vi "XIPIN_Aurora_8B10B_11_0.vi"   [LabVIEW 2017]
doc: "Customizable multi-lane gigabit serial link implementing the Aurora 8B10B protocol\n------------------------------------\n<b>Need License</b> : No\n<b>Interface</b> : AXI4-Stream"
uses:
  <vilib>/rvi/XilinxIP/XIPIN_XNode/niFpgaXIPIN.xnode
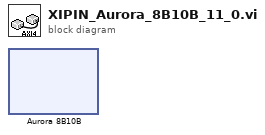
[diagram p0: block diagram]
diagram:
  n1 = xnode ("Aurora 8B10B")() -> ()
